vi "Start PID.vi"(4 "Reset PID en entrée":bool, 6 "dt (s) PID":dbl=-1.0 format="%#_13g", 7 "Centroid Variable":dbl format="%.2f", 8 "entrée d'erreur (pas d'erreur)":errorcluster, 9 "PID gains":T1={"proportional gain (Kc)"=0.7, "integral time (Ti, min)"=0.04, "derivative time (Td, min)"=0.0}, 10 "Switch Axe":bool, 11 "Refnum de .NET en entrée":refnum<k24>) -> (0 "sortie d'erreur":errorcluster, 2 "Tension Sortie PID":dbl(graph), 3 "Refnum de .NET en sortie":refnum<k24>)   [LabVIEW 2026]
uses:
  <vilib>/addons/control/pid/NI_PID_pid.lvlib
  <vilib>/addons/control/pid/pid.llb/PID (DBL).vi
  C:/Users/flepetit/Desktop/Projet BTS Photonique/Thorlabs.MotionControl.TCube.PiezoCLI.dll
  Thorlabs.MotionControl.TCube.PiezoCLI.dll
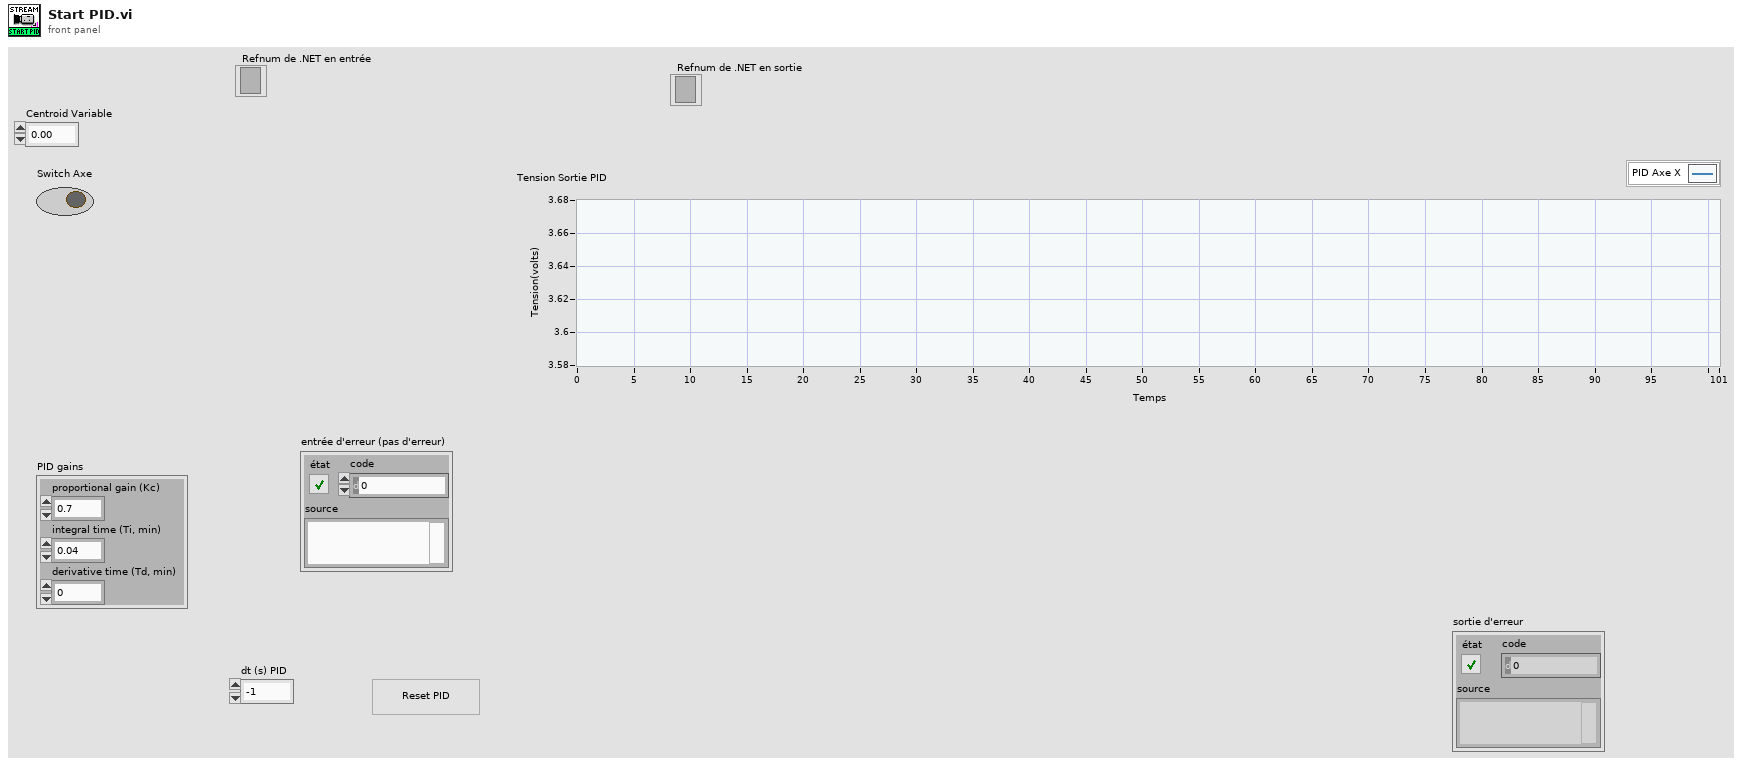
[diagram p1: front panel]
types:
  T1 = cluster{"proportional gain (Kc)":dbl, "integral time (Ti, min)":dbl, "derivative time (Td, min)":dbl}
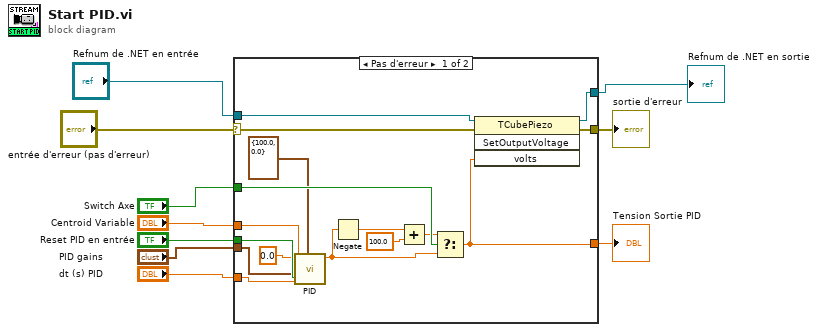
[diagram p0: block diagram]
diagram:
  n1 = case shown="Pas d'erreur" "entrée d'erreur (pas d'erreur)" {
    selector: "entrée d'erreur (pas d'erreur)" -> [w12 w28]
    tunnel: "dt (s) PID" -> [w26 _]
    tunnel: [w25 _] -> w9
    tunnel: "Reset PID en entrée" -> [w24 _]
    tunnel: "Switch Axe" -> [w23 _]
    tunnel: "PID gains" -> [w18 _]
    tunnel: "Refnum de .NET en entrée" -> [w15 w27]
    tunnel: [w14 w28] -> w4
    tunnel: "Centroid Variable" -> [w13 _]
    tunnel: [w11 w27] -> w1
    frame No Error {
      n2 = call-poly <vilib>:"PID.vi"("reinitialize? (F)"=w24, "output range"=cluster{"output high":dbl, "output low":dbl} {"output high"=100.0, "output low"=0.0}, "dt (s)"=w26, "PID gains"=w18, "process variable"=w13, "setpoint"=0.0) -> ("output"=w22:dbl)  [unwired: 4 in, 1 out]
      n3 = Negate(x=w22) -> (-x=w21:dbl)
      n4 = Add(x=w21, y=100.0 ("output high")) -> (x+y=w19:dbl)
      n5 = Select(t=w19, s=w23, f=w22) -> (s? t:f=w25:dbl)
      n6 = invoke class="TCubePiezo" method="SetOutputVoltage"(reference=w15, error in=w12, "volts"=w25) -> (reference out=w11:refnum<k24>, error out=w14:errorcluster)  [unwired: 1 in, 2 out]
    }
    frame Error {
    }
  }
  "Tension Sortie PID" <- w9
  "sortie d'erreur" <- w4
  "Refnum de .NET en sortie" <- w1
